vi "getDIO.vi"(8 "error in (no error)":errorcluster) -> (0 "error out":errorcluster, 3 "DIO state":T1)   [LabVIEW 2010, in "TPVG_DLL.lvlib"]
doc: "get DIO config information and state\n------------------------------------------\nAuthor: Dang Lam\nEmail: danglamtd@gmail.com"
uses:
  TPVG_DLL.lvlib
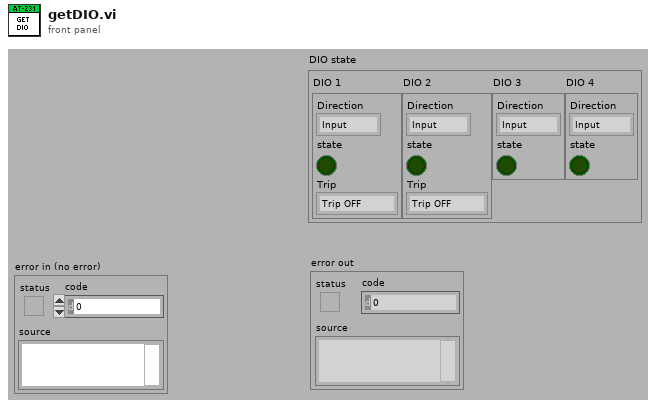
[diagram p1: front panel]
types:
  T1 = cluster{"DIO 1":cluster{"Direction":enum16{"Input", "Output"}, "state":bool, "Trip":enum16{"Trip OFF", "Trip ON"}}, "DIO 2":cluster{"Direction":enum16{"Input", "Output"}, "state":bool, "Trip":enum16{"Trip OFF", "Trip ON"}}, "DIO 3":cluster{"Direction":enum16{"Input", "Output"}, "state":bool}, "DIO 4":cluster{"Direction":enum16{"Input", "Output"}, "state":bool}}
  T2 = cluster{"Direction":enum16{"Input", "Output"}, bool}
  T3 = cluster{"Direction":enum16{"Input", "Output"}, bool, "Trip":enum16{"Trip OFF", "Trip ON"}}
  T4 = cluster{cluster{"Direction":enum16{"Input", "Output"}, bool, "Trip":enum16{"Trip OFF", "Trip ON"}}, cluster{"Direction":enum16{"Input", "Output"}, bool, "Trip":enum16{"Trip OFF", "Trip ON"}}, cluster{"Direction":enum16{"Input", "Output"}, bool}, cluster{"Direction":enum16{"Input", "Output"}, bool}}
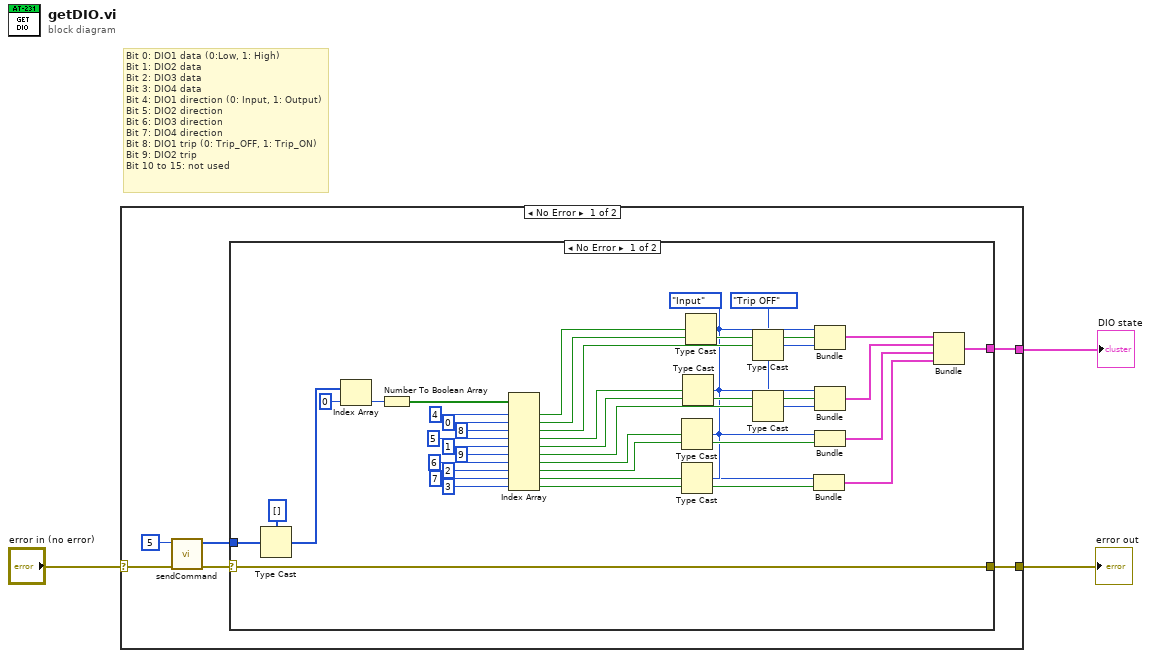
[diagram p0: block diagram]
diagram:
  # "Bit 0: DIO1 data (0:Low, 1: High)\nBit 1: DIO2 data\nBit 2: DIO3 data\nBit 3: DIO4 data\nBit 4: DIO1 direction (0: Input, 1: Output)\nBit 5: DIO2 direction\nBit 6: DIO3 direction\nBit 7: DIO4 direction\nBit 8: DIO1 trip (0: Trip_OFF, 1: Trip_ON)\nBit 9: DIO2 trip\nBit 10 to 15: not used"
  n1 = case shown="No Error" "error in (no error)" {
    selector: "error in (no error)" -> [w9 w51]
    tunnel: [w6 w51] -> w2
    tunnel: [w4 _] -> w1
    frame No Error {
      n2 = call "sendCommand.vi"("error in (no error)"=w9, "Command ID"=u16 5) -> ("error out"=w7:errorcluster, "Data out"=w5:u8[])  [unwired: 8 in]
      n3 = case shown="No Error" w7 {
        selector: w7 -> [w49 w50]
        tunnel: [w49 w50] -> w6
        tunnel: w5 -> [w48 _]
        tunnel: [w10 _] -> w4
        frame No Error {
          w24 = enum16{"Trip OFF", "Trip ON"}."Trip OFF" ("Trip")
          w18 = enum16{"Input", "Output"}."Input" ("Direction")
          n4 = Type Cast(type=u16[] [], x=w48) -> (*(type *) &x=w46:u16[])
          n5 = Index Array(array=w46, index=0) -> (element=w44:u16)
          n6 = Number To Boolean Array(number=w44) -> (Boolean array=w43:bool[])
          n7 = Index Array(array=w43, index #1=4 ("index"), index #2=0 ("index"), index #3=8 ("index"), index #4=5 ("index"), index #5=1 ("index"), index #6=9 ("index"), index #7=6 ("index"), index #8=2 ("index"), index #9=7 ("index"), index #10=3 ("index")) -> (element #1=w32:bool, element #2=w30:bool, element #3=w29:bool, element #4=w27:bool, element #5=w25:bool, element #6=w23:bool, element #7=w21:bool, element #8=w19:bool, element #9=w17:bool, element #10=w15:bool)
          n8 = Type Cast(type=w18, x=w21) -> (*(type *) &x=w20:enum16{"Input", "Output"})
          n9 = Type Cast(type=w18, x=w17) -> (*(type *) &x=w16:enum16{"Input", "Output"})
          n10 = Type Cast(type=w18, x=w27) -> (*(type *) &x=w26:enum16{"Input", "Output"})
          n11 = Type Cast(type=w18, x=w32) -> (*(type *) &x=w31:enum16{"Input", "Output"})
          n12 = Type Cast(type=w24, x=w29) -> (*(type *) &x=w28:enum16{"Trip OFF", "Trip ON"})
          n13 = Type Cast(type=w24, x=w23) -> (*(type *) &x=w22:enum16{"Trip OFF", "Trip ON"})
          n14 = Bundle("Direction"=w16, w15) -> (w11:T2)  [unwired: 1 in]
          n15 = Bundle("Direction"=w31, w30, "Trip"=w28) -> (w14:T3)  [unwired: 1 in]
          n16 = Bundle("Direction"=w26, w25, "Trip"=w22) -> (w13:T3)  [unwired: 1 in]
          n17 = Bundle("Direction"=w20, w19) -> (w12:T2)  [unwired: 1 in]
          n18 = Bundle(w14, w13, w12, w11) -> (w10:T4)  [unwired: 1 in]
        }
        frame Error {
        }
      }
    }
    frame Error {
    }
  }
  "error out" <- w2
  "DIO state" <- w1
